vi "Heater_Safety.vi"(6 "Ch Names":string[](array[string]), 7 "Values":dbl[](array[numeric]) format="%.2f") -> (1 "Error String":string)   [LabVIEW 2020]
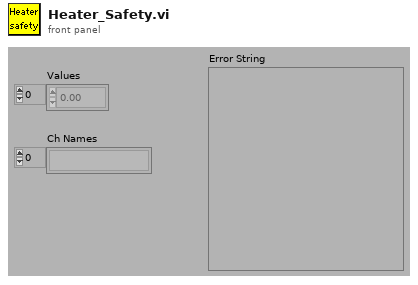
[diagram p1: front panel]
types:
  T1 = typedef "Ch_description_ADAM.ctl" = cluster{"Ch Name":string, "Type":T2, "Function":T3, "Ch State":T4, "Calibration type":T5, "A":dbl, "B":dbl, "C":dbl, "D":dbl, "Comments":string, "Address":T6, "String":string, "Duty":u16}
  T2 = typedef "Module_type_ADAM.ctl" = string
  T3 = typedef "Function_ADAM.ctl" = enum16{"Analogue Input", "Digital Input", "Event counter", "Event rate", "Analogue Output", "Digital Output", "Relay Output"}
  T4 = typedef "Channel_State.ctl" = enum16{"On", "Off", "Always On", "Always Off"}
  T5 = typedef "Calib_type_ADAM.ctl" = string
  T6 = typedef "Address.ctl" = cluster{"Main":i32, "Ch.":i32, "Sub":i32, "Port Name":string}
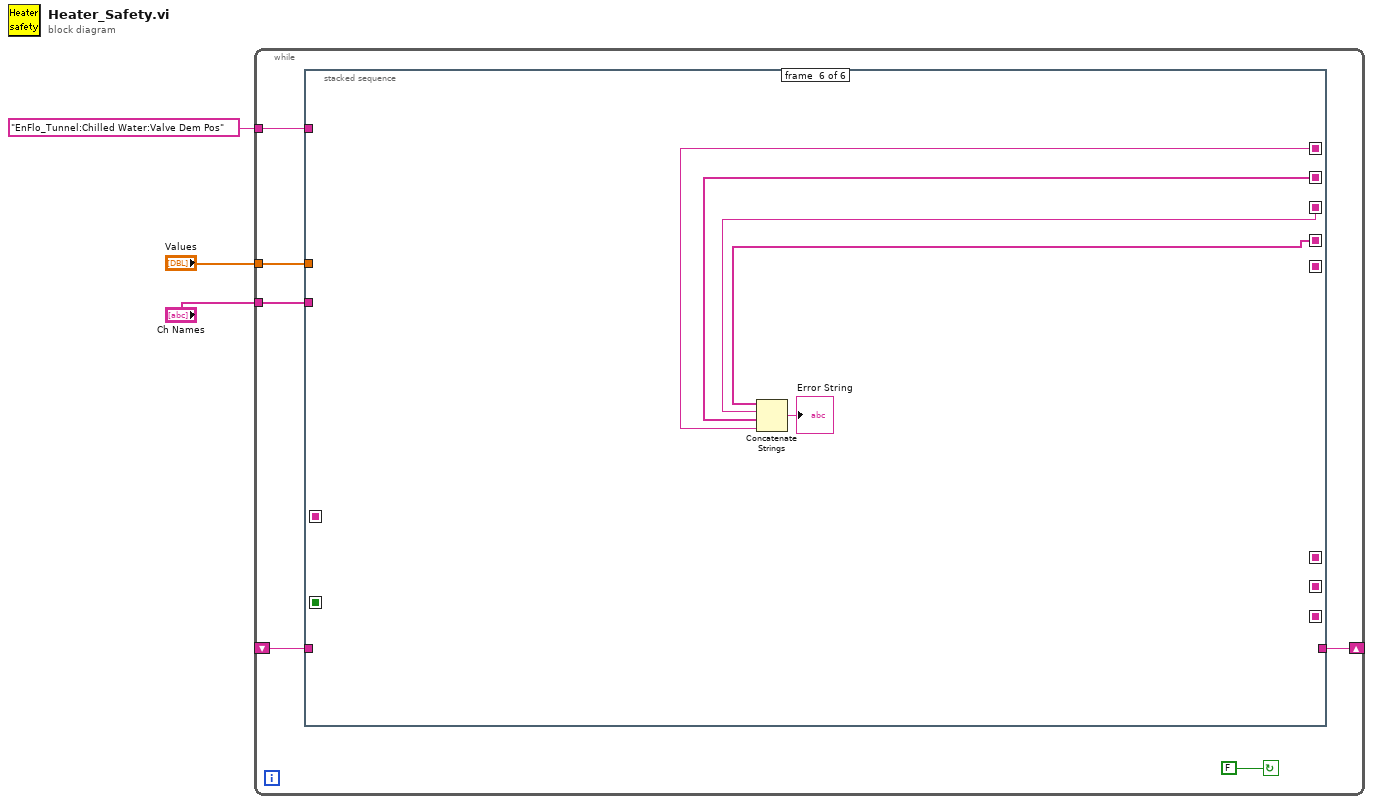
[diagram p0: block diagram]
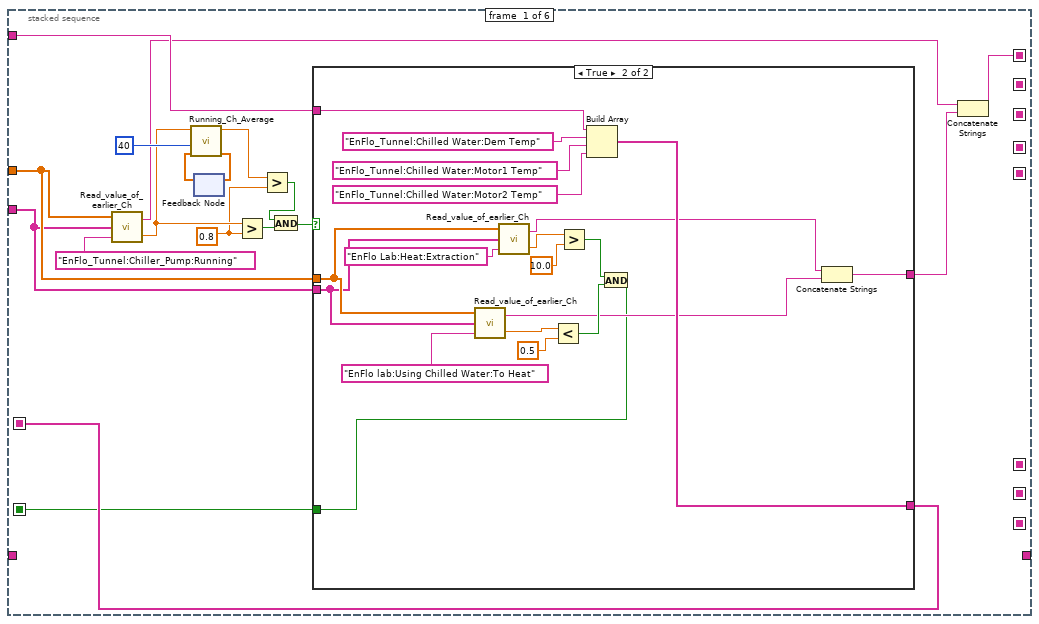
[diagram p2: hidden frame]
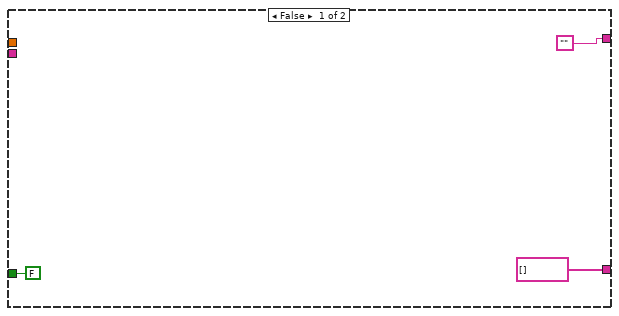
[diagram p3: hidden frame]
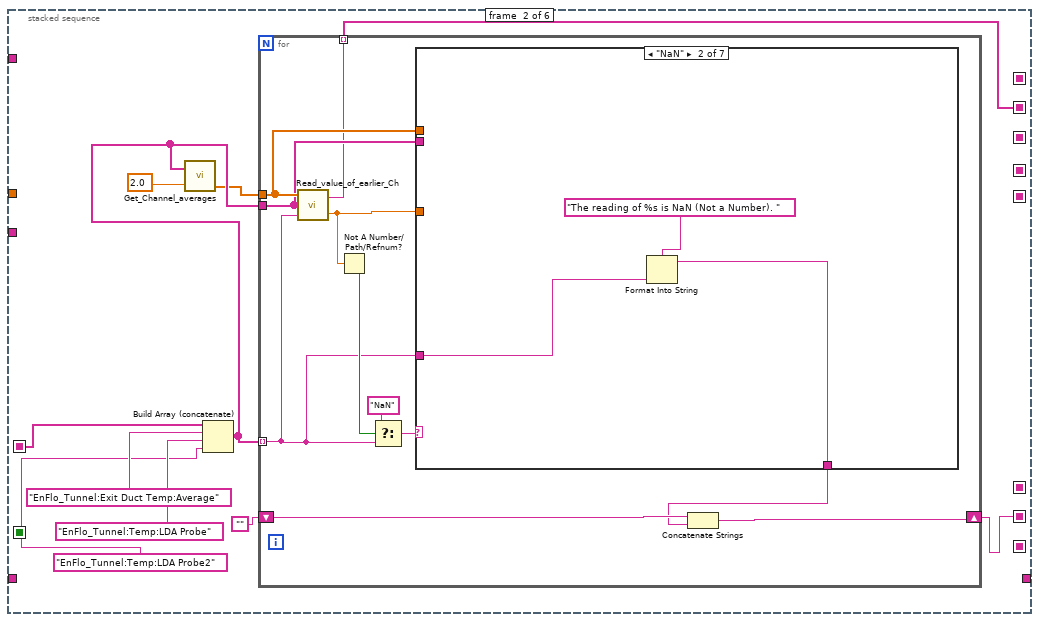
[diagram p4: hidden frame]
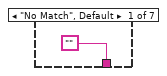
[diagram p5: hidden frame]
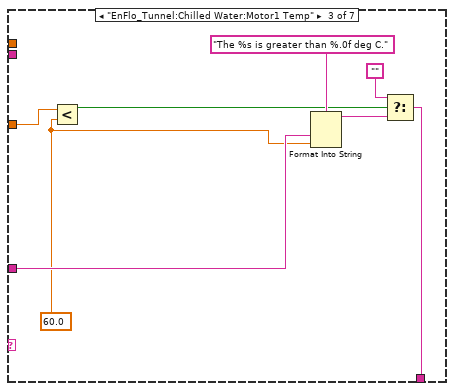
[diagram p6: hidden frame]
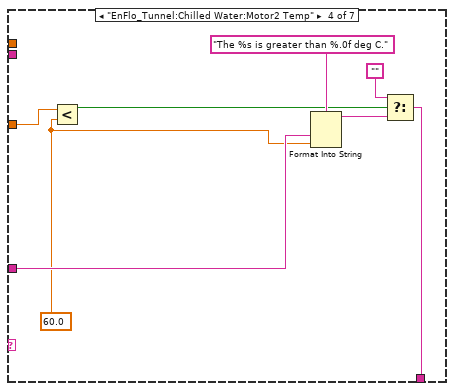
[diagram p7: hidden frame]
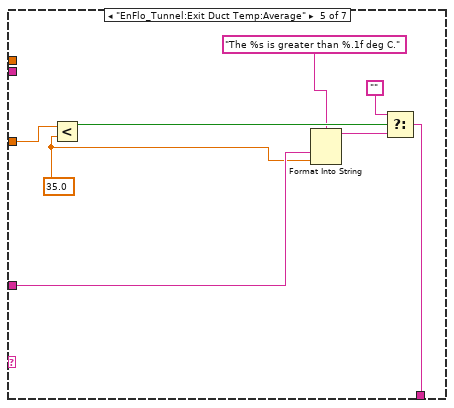
[diagram p8: hidden frame]
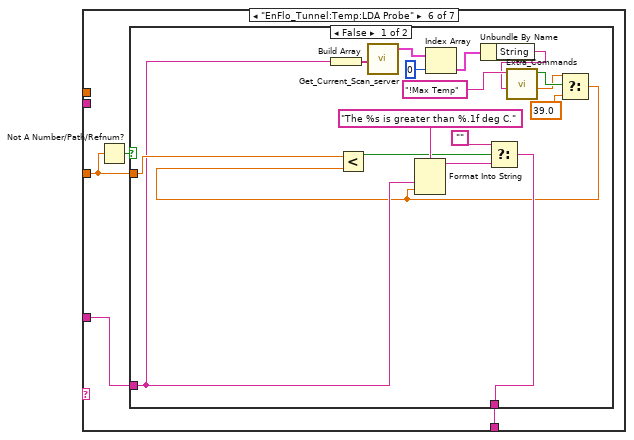
[diagram p9: hidden frame]
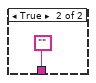
[diagram p10: hidden frame]
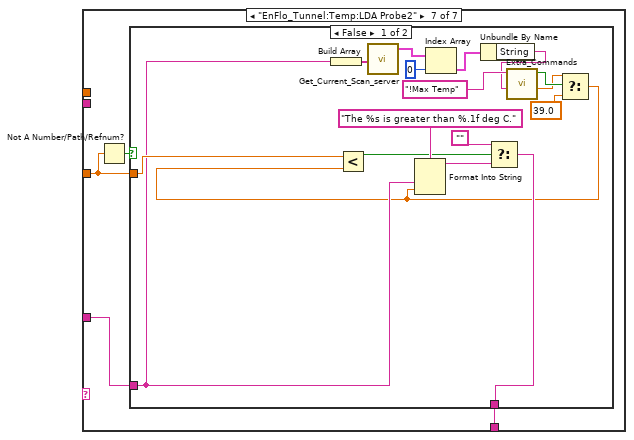
[diagram p11: hidden frame]
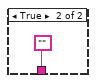
[diagram p12: hidden frame]
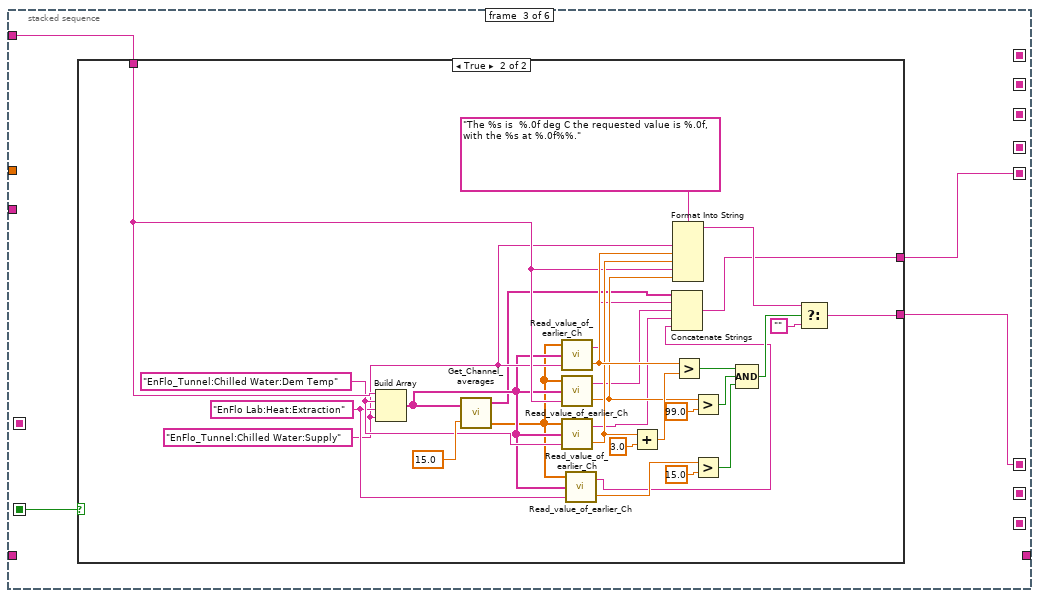
[diagram p13: hidden frame]
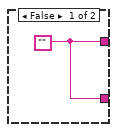
[diagram p14: hidden frame]
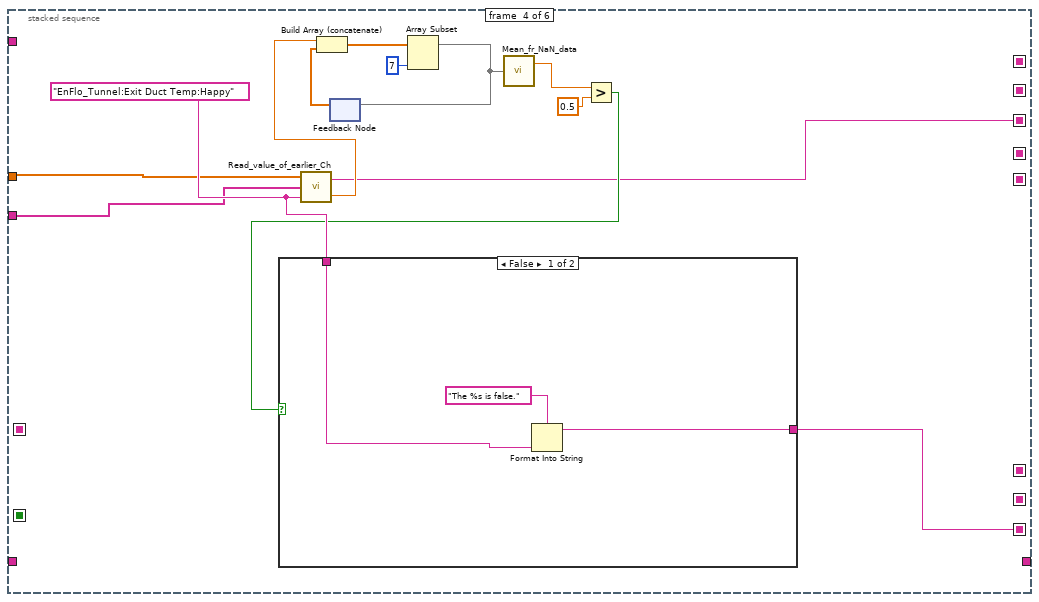
[diagram p15: hidden frame]
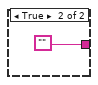
[diagram p16: hidden frame]
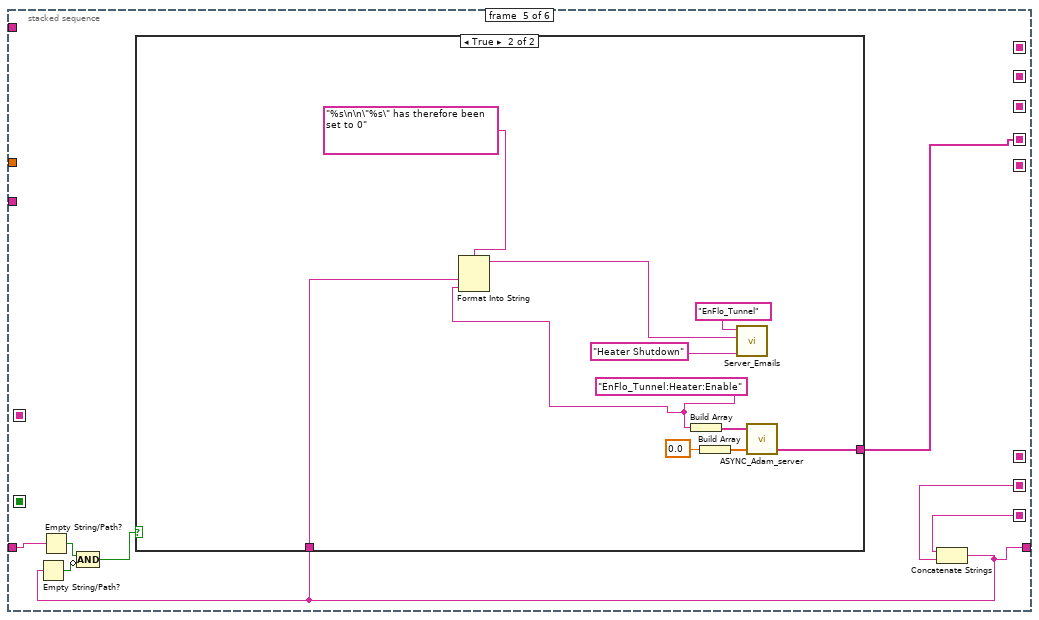
[diagram p17: hidden frame]
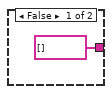
[diagram p18: hidden frame]
diagram:
  n1 = while {
    shift-left: _ -> [w7]
    shift-right: [w8] -> _
    tunnel: "Values" -> [w6]
    tunnel: "Ch Names" -> [w5]
    tunnel: "EnFlo_Tunnel:Chilled Water:Valve Dem Pos" -> [w4]
    stop <- FALSE continue-if-true
    n2 = stacked-sequence {
      seq-local: [_ w54 _ _ _ _] -> [_ _ _ _ w196 _]
      seq-local: [w26 _ _ _ _ _] -> [_ w52 _ _ _ _]
      seq-local: [_ _ _ w181 _ _] -> [_ _ _ _ w197 _]
      seq-local: [w12 _ _ _ _ _] -> [_ _ _ _ _ w214]
      seq-local: [_ w50 _ _ _ _] -> [_ _ _ _ _ w215]
      seq-local: [_ _ _ w179 _ _] -> [_ _ _ _ _ w216]
      seq-local: [_ _ _ _ w194 _] -> [_ _ _ _ _ w217]
      seq-local: [_ _ w144 _ _ _] -> [_ _ _ _ _ _]
      seq-local: [_ _ w146 _ _ _] -> [_ _ _ _ _ _]
      seq-local: [w10 _ _ _ _ _] -> [_ _ w143 _ _ _]
      tunnel: [_ _ _ _ w195 _] -> w8
      tunnel: w7 -> [_ _ _ _ w201 _]
      tunnel: w6 -> [w25 _ _ w183 _ _]
      tunnel: w5 -> [w24 _ _ w182 _ _]
      tunnel: w4 -> [w23 _ w145 _ _ _]
      frame #0 {
        w14 = 0.8 ("y")
        n3 = call "Read_value_of_earlier_Ch.vi"("Desired Ch to Read"="EnFlo_Tunnel:Chiller_Pump:Running", "Ch names"=w24, "Present scan array"=w25) -> ("Value"=w19:dbl, "Scan comment"=w11:string)  [unwired: 1 in]
        n4 = feedback #1() -> (w21:dbl[])  [unwired: 1 in]
        n5 = call "Running_Ch_Average.vi"("Shift In"=w21, "History length"=40, "New Value"=w19) -> ("Shift Out"=w22:dbl[], "mean"=w18:dbl)  [unwired: 2 in, 1 out]
        n6 = feedback-in #1(w22) -> ()
        n7 = Greater?(x=w19, y=w14) -> (0:w16:bool)
        n8 = Greater?(x=w18, y=w14) -> (0:w17:bool)
        n9 = And(x=w17, y=w16) -> (x .and. y?=w15:bool)
        n10 = case shown="True" w15 {
          tunnel: [string[] [] w45] -> w26
          tunnel: w25 -> [_ w44]
          tunnel: w24 -> [_ w43]
          tunnel: w23 -> [_ w38]
          tunnel: ["" w32] -> w13
          tunnel: [FALSE w31] -> w10
          frame False {
          }
          frame True {
            n11 = call "Read_value_of_earlier_Ch.vi"("Desired Ch to Read"="EnFlo lab:Using Chilled Water:To Heat", "Ch names"=w43, "Present scan array"=w44) -> ("Value"=w37:dbl, "Scan comment"=w33:string)  [unwired: 1 in]
            n12 = call "Read_value_of_earlier_Ch.vi"("Desired Ch to Read"="EnFlo Lab:Heat:Extraction", "Ch names"=w43, "Present scan array"=w44) -> ("Value"=w41:dbl, "Scan comment"=w34:string)  [unwired: 1 in]
            n13 = Less?(x=w37, y=0.5) -> (x < y?=w35:bool)
            n14 = Greater?(x=w41, y=10.0) -> (0:w39:bool)
            n15 = Build Array(w38, "EnFlo_Tunnel:Chilled Water:Dem Temp", "EnFlo_Tunnel:Chilled Water:Motor1 Temp", "EnFlo_Tunnel:Chilled Water:Motor2 Temp") -> (w45:string[])
            n16 = And(x=w39, y=w35) -> (x .and. y?=w31:bool)
            n17 = Concatenate Strings(w34, w33) -> (w32:string)
          }
        }
        n18 = Concatenate Strings(w11, w13) -> (w12:string)
      }
      frame #1 {
        n19 = Build Array (concatenate)(w52, "EnFlo_Tunnel:Exit Duct Temp:Average", "EnFlo_Tunnel:Temp:LDA Probe", "EnFlo_Tunnel:Temp:LDA Probe2") -> (w58:string[])
        n20 = call "Get_Channel_averages.vi"("Desired Ch Names"=w58, "Averaging time (mins)"=2.0) -> ("number"=w55:dbl[])  [unwired: 1 in, 2 out]
        n21 = for {
          tunnel: w58 -> [w61]
          tunnel: w55 -> [w62]
          tunnel: w58 -> [w64] mode=indexing
          shift-right: [w69] -> w54
          shift-left: "" -> [w70]
          tunnel: [w60] -> w50 mode=indexing
          n22 = call "Read_value_of_earlier_Ch.vi"("Desired Ch to Read"=w64, "Ch names"=w61, "Present scan array"=w62) -> ("Value"=w67:dbl, "Scan comment"=w60:string)  [unwired: 1 in]
          n23 = Not A Number/Path/Refnum?(number/path/refnum=w67) -> (NaN/Path/Refnum?=w66:bool)
          n24 = Select(t="NaN", s=w66, f=w64) -> (s? t:f=w63:string)
          n25 = case shown="\"NaN\"" w63 {
            tunnel: w67 -> [_ _ w82 w90 w94 w100 w122]
            tunnel: w64 -> [_ w72 w81 w89 w98 w102 w124]
            tunnel: ["" w73 w75 w83 w95 w101 w123] -> w68
            tunnel: w62 -> [_ _ _ _ _ _ _]
            tunnel: w61 -> [_ _ _ _ _ _ _]
            frame "No Match", Default {
            }
            frame "NaN" {
              n26 = Format Into String(format string="The reading of %s is NaN (Not a Number). " ("Format String"), w72) -> (resulting string=w73:string)  [unwired: 2 in, 1 out]
            }
            frame "EnFlo_Tunnel:Chilled Water:Motor1 Temp" {
              w80 = 60.0 ("y")
              n27 = Less?(x=w82, y=w80) -> (x < y?=w78:bool)
              n28 = Format Into String(format string="The %s is greater than %.0f deg C." ("Format String"), w81, w80) -> (resulting string=w77:string)  [unwired: 2 in, 1 out]
              n29 = Select(t="", s=w78, f=w77) -> (s? t:f=w75:string)
            }
            frame "EnFlo_Tunnel:Chilled Water:Motor2 Temp" {
              w88 = 60.0 ("y")
              n30 = Less?(x=w90, y=w88) -> (x < y?=w86:bool)
              n31 = Format Into String(format string="The %s is greater than %.0f deg C." ("Format String"), w89, w88) -> (resulting string=w85:string)  [unwired: 2 in, 1 out]
              n32 = Select(t="", s=w86, f=w85) -> (s? t:f=w83:string)
            }
            frame "EnFlo_Tunnel:Exit Duct Temp:Average" {
              w97 = 35.0 ("y")
              n33 = Less?(x=w94, y=w97) -> (x < y?=w96:bool)
              n34 = Format Into String(format string="The %s is greater than %.1f deg C." ("Format String"), w98, w97) -> (resulting string=w92:string)  [unwired: 2 in, 1 out]
              n35 = Select(t="", s=w96, f=w92) -> (s? t:f=w95:string)
            }
            frame "EnFlo_Tunnel:Temp:LDA Probe" {
              n36 = Not A Number/Path/Refnum?(number/path/refnum=w100) -> (NaN/Path/Refnum?=w99:bool)
              n37 = case shown="False" w99 {
                tunnel: w100 -> [w119 _]
                tunnel: w102 -> [w113 _]
                tunnel: [w114 ""] -> w101
                frame False {
                  n38 = Build Array(w113) -> (w112:string[])
                  n39 = call "Get_Current_Scan_server.vi"("Desired Channels"=w112) -> ("Ch Description Array"=w111:T1[])  [unwired: 2 out]
                  n40 = Index Array(array=w111, index=0 ("Index")) -> (element=w109:T1)
                  n41 = Unbundle By Name(w109) -> ("String"=w103:string)
                  n42 = call "Extra_Commands.vi"("String to Search"=w103, "Command"="!Max Temp") -> ("Numeric Value"=w106:dbl, "Command Found"=w107:bool)  [unwired: 1 in, 3 out]
                  n43 = Select(t=w106, s=w107, f=39.0) -> (s? t:f=w104:dbl)
                  n44 = Less?(x=w119, y=w104) -> (x < y?=w115:bool)
                  n45 = Format Into String(format string="The %s is greater than %.1f deg C." ("Format String"), w113, w104) -> (resulting string=w117:string)  [unwired: 2 in, 1 out]
                  n46 = Select(t="", s=w115, f=w117) -> (s? t:f=w114:string)
                }
                frame True {
                }
              }
            }
            frame "EnFlo_Tunnel:Temp:LDA Probe2" {
              n47 = Not A Number/Path/Refnum?(number/path/refnum=w122) -> (NaN/Path/Refnum?=w121:bool)
              n48 = case shown="False" w121 {
                tunnel: w122 -> [w141 _]
                tunnel: w124 -> [w135 _]
                tunnel: [w136 ""] -> w123
                frame False {
                  n49 = Build Array(w135) -> (w134:string[])
                  n50 = call "Get_Current_Scan_server.vi"("Desired Channels"=w134) -> ("Ch Description Array"=w133:T1[])  [unwired: 2 out]
                  n51 = Index Array(array=w133, index=0 ("Index")) -> (element=w131:T1)
                  n52 = Unbundle By Name(w131) -> ("String"=w125:string)
                  n53 = call "Extra_Commands.vi"("String to Search"=w125, "Command"="!Max Temp") -> ("Numeric Value"=w128:dbl, "Command Found"=w129:bool)  [unwired: 1 in, 3 out]
                  n54 = Select(t=w128, s=w129, f=39.0) -> (s? t:f=w126:dbl)
                  n55 = Less?(x=w141, y=w126) -> (x < y?=w137:bool)
                  n56 = Format Into String(format string="The %s is greater than %.1f deg C." ("Format String"), w135, w126) -> (resulting string=w139:string)  [unwired: 2 in, 1 out]
                  n57 = Select(t="", s=w137, f=w139) -> (s? t:f=w136:string)
                }
                frame True {
                }
              }
            }
          }
          n58 = Concatenate Strings(w70, w68) -> (w69:string)
        }
      }
      frame #2 {
        n59 = case shown="True" w143 {
          tunnel: [w147 w160] -> w146
          tunnel: w145 -> [_ w159]
          tunnel: [w147 w148] -> w144
          frame False {
            w147 = ""
          }
          frame True {
            w156 = "EnFlo_Tunnel:Chilled Water:Supply"
            w157 = "EnFlo Lab:Heat:Extraction" ("Desired Ch to Read")
            w158 = "EnFlo_Tunnel:Chilled Water:Dem Temp"
            n60 = Build Array(w159, w158, w157, w156) -> (w155:string[])
            n61 = call "Get_Channel_averages.vi"("Desired Ch Names"=w155, "Averaging time (mins)"=15.0) -> ("Comments"=w153:string[], "number"=w154:dbl[])  [unwired: 1 in, 1 out]
            n62 = call "Read_value_of_earlier_Ch.vi"("Desired Ch to Read"=w156, "Ch names"=w155, "Present scan array"=w154) -> ("Value"=w175:dbl, "Scan comment"=w152:string)  [unwired: 1 in]
            n63 = call "Read_value_of_earlier_Ch.vi"("Desired Ch to Read"=w159, "Ch names"=w155, "Present scan array"=w154) -> ("Value"=w164:dbl, "Scan comment"=w151:string)  [unwired: 1 in]
            n64 = call "Read_value_of_earlier_Ch.vi"("Desired Ch to Read"=w158, "Ch names"=w155, "Present scan array"=w154) -> ("Value"=w165:dbl, "Scan comment"=w150:string)  [unwired: 1 in]
            n65 = call "Read_value_of_earlier_Ch.vi"("Desired Ch to Read"=w157, "Ch names"=w155, "Present scan array"=w154) -> ("Value"=w163:dbl, "Scan comment"=w149:string)  [unwired: 1 in]
            n66 = Add(x=w165, y=3.0) -> (x+y=w166:dbl)
            n67 = Concatenate Strings(w153, w152, w151, w150, w149) -> (w148:string)
            n68 = Format Into String(format string="The %s is  %.0f deg C the requested value is %.0f, with the %s at %.0f%%." ("Format String"), w156, w175, w165, w159, w164) -> (resulting string=w168:string)  [unwired: 2 in, 1 out]
            n69 = Greater?(x=w175, y=w166) -> (0:w170:bool)
            n70 = Greater?(x=w164, y=99.0) -> (0:w171:bool)
            n71 = Greater?(x=w163, y=15.0) -> (0:w161:bool)
            n72 = Compound Arithmetic op=AND(w170, w171, w161) -> (w169:bool)
            n73 = Select(t=w168, s=w169, f="") -> (s? t:f=w160:string)
          }
        }
      }
      frame #3 {
        w189 = "EnFlo_Tunnel:Exit Duct Temp:Happy" ("Desired Ch to Read")
        n74 = call "Read_value_of_earlier_Ch.vi"("Desired Ch to Read"=w189, "Ch names"=w182, "Present scan array"=w183) -> ("Value"=w188:dbl, "Scan comment"=w179:string)  [unwired: 1 in]
        n75 = feedback #2() -> (w186:dbl[])  [unwired: 1 in]
        n76 = Build Array (concatenate)(w188, w186) -> (w185:dbl[])
        n77 = Array Subset(array=w185, length=7) -> (w178:dbl[])  [unwired: 1 in]
        n78 = feedback-in #2(w178) -> ()
        n79 = call "Mean_fr_NaN_data.vi"("Data"=w178) -> ("Mean value"=w177:dbl)  [unwired: 1 out]
        n80 = Greater?(x=w177, y=0.5) -> (0:w180:bool)
        n81 = case shown="False" w180 {
          tunnel: w189 -> [w192 _]
          tunnel: [w190 ""] -> w181
          frame False {
            n82 = Format Into String(format string="The %s is false.", w192) -> (resulting string=w190:string)  [unwired: 2 in, 1 out]
          }
          frame True {
          }
        }
      }
      frame #4 {
        n83 = Empty String/Path?(string/path=w201) -> (empty?=w200:bool)
        n84 = Concatenate Strings(w197, w196) -> (w195:string)
        n85 = Empty String/Path?(string/path=w195) -> (empty?=w199:bool)
        n86 = Compound Arithmetic op=AND(w200, invert w199) -> (w198:bool)
        n87 = case shown="True" w198 {
          tunnel: w195 -> [_ w205]
          tunnel: [string[] [] ("Scan Comments") w203] -> w194
          frame False {
          }
          frame True {
            w206 = "EnFlo_Tunnel:Heater:Enable"
            n88 = Format Into String(format string="%s\n\n\"%s\" has therefore been set to 0", w205, w206) -> (resulting string=w204:string)  [unwired: 2 in, 1 out]
            n89 = Build Array(w206) -> (w207:string[])
            n90 = Build Array(0.0) -> (w208:dbl[])
            n91 = call "Server_Emails.vi"("Client Name Contains"="EnFlo_Tunnel", "Message"=w204, "Subject"="Heater Shutdown" ("t")) -> ()  [unwired: 2 in, 3 out]
            n92 = call "ASYNC_Adam_server.vi"("Values"=w208, "Channel Names"=w207) -> ("Scan Comments"=w203:string[])  [unwired: 1 in, 2 out]
          }
        }
      }
      frame #5 {
        n93 = Concatenate Strings(w217, w216, w215, w214) -> (→"Error String":string)
      }
    }
  }
